vi "Jog.vi"(8 "error in (no error)":errorcluster, 9 "Step size":dbl, 10 "Direction":enum16{"Right", "Left", "Up", "Down"}(ring), 11 "Microscope":refnum<class "Microscope.lvclass">) -> (0 "error out":errorcluster, 3 "Microscope out":refnum<class "Microscope.lvclass">)   [LabVIEW 2015, in "Microscope.lvclass"]
doc: "---------------------------------------------------------------\nJKI State Machine Objects™\nhttp://jki.net/state-machine-objects/\nCopyright (C) 2005-2015, JKI <info@jki.net>\nALL RIGHTS RESERVEDJKI State Machine Objects (SMO) 1.0.0.4\nJKI - JKI\nCopyright (c) 2015, JKI"
uses:
  Microscope.lvclass
  XYStage/Typedefs/(real)Coords--Cluster.ctl
  XYStage/XYStage.lvclass
panel:
  # "For instructions on how to use the JKI State Machine Objects, examples and video tutorials, visit:\nhttp://jki.net/state-machine-objects/\n\nJKI State Machine Objects™\nhttp://jki.net/state-machine-objects/\nCopyright (C) 2005-2015, JKI <info@jki.net>\nALL RIGHTS RESERVED"
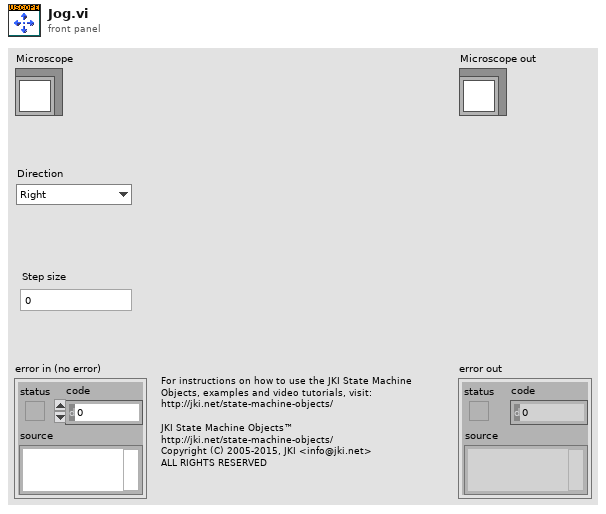
[diagram p1: front panel]
types:
  T1 = typedef "XYStage.lvclass/(real)Coords--Cluster.ctl" = cluster{"X":dbl, "Y":dbl}
  T2 = typedef "Microscope.lvclass/Dependencies--Cluster.ctl" = cluster{"XYStage":refnum<class "XYStage.lvclass">, "Camera":refnum<class "Camera.lvclass">}
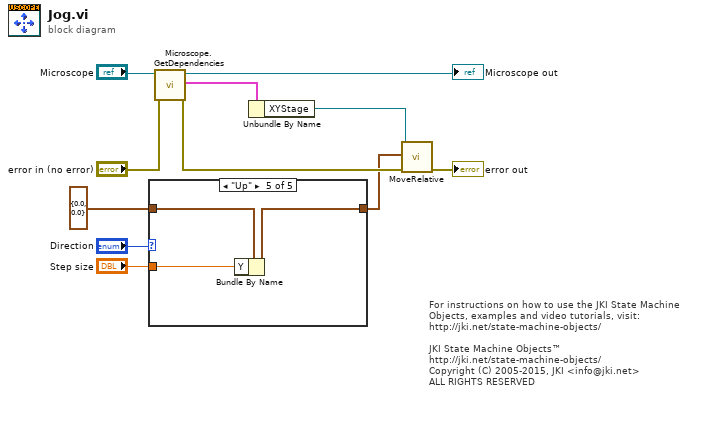
[diagram p0: block diagram]
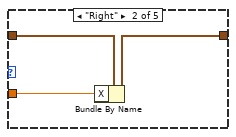
[diagram p3: hidden frame]
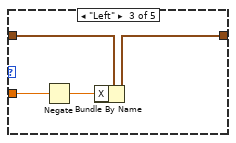
[diagram p4: hidden frame]
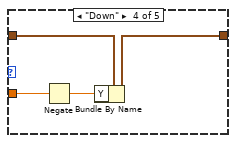
[diagram p5: hidden frame]
diagram:
  # "For instructions on how to use the JKI State Machine Objects, examples and video tutorials, visit:\nhttp://jki.net/state-machine-objects/\n\nJKI State Machine Objects™\nhttp://jki.net/state-machine-objects/\nCopyright (C) 2005-2015, JKI <info@jki.net>\nALL RIGHTS RESERVED"
  n1 = case shown="\"Up\"" "Direction" {
    tunnel: T1 {"X"=0.0, "Y"=0.0} ("Units") -> [w12 w15 w19 w23 w26]
    tunnel: [w12 w13 w17 w21 w25] -> w2
    tunnel: "Step size" -> [_ w14 w18 w22 w24]
    frame Default {
    }
    frame "Right" {
      n2 = Bundle By Name(cluster=w15, "X"=w14) -> (w13:T1)
    }
    frame "Left" {
      n3 = Negate(x=w18) -> (-x=w16:dbl)
      n4 = Bundle By Name(cluster=w19, "X"=w16) -> (w17:T1)
    }
    frame "Down" {
      n5 = Negate(x=w22) -> (-x=w20:dbl)
      n6 = Bundle By Name(cluster=w23, "Y"=w20) -> (w21:T1)
    }
    frame "Up" {
      n7 = Bundle By Name(cluster=w26, "Y"=w24) -> (w25:T1)
    }
  }
  n8 = call "Microscope.GetDependencies.vi"("error in (no error)"="error in (no error)", "Microscope"="Microscope") -> ("error out"=w6:errorcluster, "Dependencies"=w8:T2, "Microscope out"=→"Microscope out":refnum<class "Microscope.lvclass">)  [unwired: 7 in]
  n9 = Unbundle By Name(w8) -> ("XYStage"=w7:refnum<class "XYStage.lvclass">)
  n10 = call "MoveRelative.vi"("error in (no error)"=w6, "Units"=w2, "XYStage"=w7) -> ("error out"=→"error out":errorcluster)  [unwired: 7 in, 1 out]
